vi "OP500Z8P_TenmaReadCurr.vi"(8 "errin":errorcluster caption="entrée d'erreur (pas d'erreur)", 11 "Visa in tenma":refnum<visa-resource-name>) -> (0 "sortie d'erreur":errorcluster, 1 "I tenma (A)":dbl, 2 "read buffer":string, 3 "In Range?":bool, 5 "cont fermés ?":bool)   [LabVIEW 2020]
uses:
  <vilib>/Instr/_visa.llb/VISA Configure Serial Port (Instr).vi
  VG/VG_TenmaParam.vi
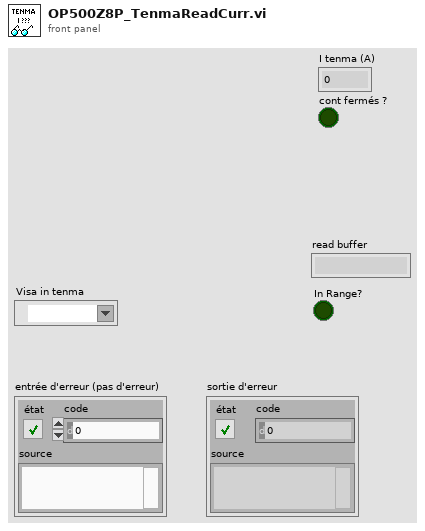
[diagram p1: front panel]
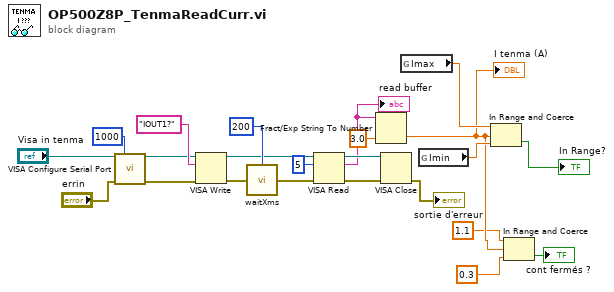
[diagram p0: block diagram]
diagram:
  n1 = call-poly "VISA Configure Serial Port"("VISA resource name"="Visa in tenma", "timeout (10sec)"=u32 1000, "error in (no error)"="errin") -> ("VISA resource name out"=w21:refnum<visa-resource-name>, "error out"=w15:errorcluster)  [unwired: 11 in]
  n2 = VISA Write(VISA resource name=w21, write buffer="IOUT1?" ("buffer d'écriture"), error in (no error)=w15) -> (VISA resource name out=w12:refnum<visa-resource-name>, error out=w20:errorcluster)  [unwired: 1 out]
  n3 = call <userlib>:"waitXms.vi"("attente (ms)"=u32 200, "errin"=w20) -> ("errout"=w14:errorcluster)  [unwired: 13 in]
  n4 = VISA Read(VISA resource name=w12, byte count=u32 5, error in (no error)=w14) -> (VISA resource name out=w10:refnum<visa-resource-name>, read buffer=w6:string, error out=w13:errorcluster)  [unwired: 1 out]
  "read buffer" <- w6
  n5 = Fract/Exp String To Number(string=w6, default (0 dbl)=3.0 ("default (0 DBL)")) -> (number=w4:dbl)  [unwired: 2 in, 1 out]
  "I tenma (A)" <- w4
  n6 = VISA Close(VISA resource name=w10, error in (no error)=w13) -> (error out=→"sortie d'erreur":errorcluster)
  n7 = global read "VG_TenmaParam.vi" "Imax"() -> (w9:dbl)
  n8 = global read "VG_TenmaParam.vi" "Imin"() -> (w8:dbl)
  n9 = In Range and Coerce(upper limit=w9, x=w4, lower limit=w8) -> (In Range?=→"In Range?":bool)  [unwired: 1 out]
  n10 = In Range and Coerce(upper limit=1.1 ("lower limit"), x=w4, lower limit=0.3 ("upper limit")) -> (In Range?=→"cont fermés ?":bool)  [unwired: 1 out]
